vi "Enqueue Error.vi"(9 "error to process":errorcluster, 10 "Error Type (Non-Critical)":T1=enum."Non-Critical Error", 11 "Message Queue":refnum<queue>) -> ()   [LabVIEW 2012, in "Message Queue.lvlib"]
uses:
  Message Queue.lvlib
  Message Cluster.ctl
  controls/Error Type.ctl
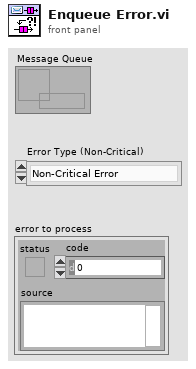
[diagram p1: front panel]
types:
  T1 = typedef "Error Type.ctl" = enum16{"Log-Only Error", "Non-Critical Error", "Critical Error"}
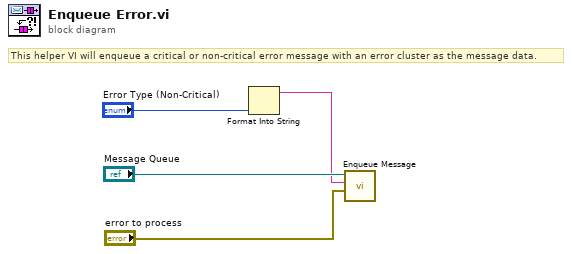
[diagram p0: block diagram]
diagram:
  # "This helper VI will enqueue a critical or non-critical error message with an error cluster as the message data."
  n1 = Format Into String("Error Type (Non-Critical)") -> (resulting string=w1:string)  [unwired: 3 in, 1 out]
  n2 = call "Enqueue Message.vi"("Message Data"="error to process", "Message"=w1, "Message Queue"="Message Queue") -> ()  [unwired: 7 in, 2 out]
